vi "sv_Weighting Network Tolerances.vi"(9 "type or class":enum16{"Type 0 / Class 1", "Type 1 / Class 2"}(ring)=enum."Type 1 / Class 2", 10 "standard":enum16{"ANSI S1.4", "IEC 61672"}(ring), 11 "frequency [Hz]":dbl=1000.0 format="%.2f") -> (2 "low tolerance [dB]":dbl format="%.2f", 3 "high tolerance [dB]":dbl format="%.2f")   [LabVIEW 2017]
panel:
  in  "IEC 61672 tolerances [dB]":T1(array[cluster])=[{"frequency [Hz]"=[10.0, 12.589254117941675, 15.848931924611142, 19.952623149688797, 25.11886431509581, 31.622776601683793, 39.810717055349734, 50.11872336272725, 63.09573444801933, 79.43282347242817, 100.0, 125.89254117941675, 158.48931924611142, 199.52623149688807, 251.18864315095823, 316.22776601683796, 398.1071705534973, 501.18723362727246, 630.9573444801937, 794.3282347242822, 1000.0, 1258.9254117941675, 1584.893192461114, 1995.262314968881, 2511.886431509582, 3162.2776601683795, 3981.0717055349733, 5011.872336272725, 6309.573444801937, 7943.282347242822, 10000.0, 12589.254117941688, 15848.93192461114, 19952.62314968879], "high limit"=[3.0, 2.5, 2.0, 2.0, 2.0, 1.5, 1.0, 1.0, 1.0, 1.0, 1.0, 1.0, 1.0, 1.0, 1.0, 1.0, 1.0, 1.0, 1.0, 1.0, 0.7, 1.0, 1.0, 1.0, 1.0, 1.0, 1.0, 1.5, 1.5, 1.5, 2.0, 2.0, 2.5, 3.0], "low limit"=[-inf, -inf, -4.0, -2.0, -1.5, -1.5, -1.0, -1.0, -1.0, -1.0, -1.0, -1.0, -1.0, -1.0, -1.0, -1.0, -1.0, -1.0, -1.0, -1.0, -0.7, -1.0, -1.0, -1.0, -1.0, -1.0, -1.0, -1.5, -2.0, -2.5, -3.0, -5.0, -16.0, -inf]}, {"frequency [Hz]"=[10.0, 12.589254117941675, 15.848931924611142, 19.952623149688797, 25.11886431509581, 31.622776601683793, 39.810717055349734, 50.11872336272725, 63.09573444801933, 79.43282347242817, 100.0, 125.89254117941675, 158.48931924611142, 199.52623149688807, 251.18864315095823, 316.22776601683796, 398.1071705534973, 501.18723362727246, 630.9573444801937, 794.3282347242822, 1000.0, 1258.9254117941675, 1584.893192461114, 1995.262314968881, 2511.886431509582, 3162.2776601683795, 3981.0717055349733, 5011.872336272725, 6309.573444801937, 7943.282347242822, 10000.0, 12589.254117941688, 15848.93192461114, 19952.62314968879], "high limit"=[5.0, 5.0, 5.0, 3.0, 3.0, 3.0, 2.0, 2.0, 2.0, 2.0, 1.5, 1.5, 1.5, 1.5, 1.5, 1.5, 1.5, 1.5, 1.5, 1.5, 1.0, 1.5, 2.0, 2.0, 2.5, 2.5, 3.0, 3.5, 4.5, 5.0, 5.0, 5.0, 5.0, 5.0], "low limit"=[-inf, -inf, -inf, -3.0, -3.0, -3.0, -2.0, -2.0, -2.0, -2.0, -1.5, -1.5, -1.5, -1.5, -1.5, -1.5, -1.5, -1.5, -1.5, -1.5, -1.0, -1.5, -2.0, -2.0, -2.5, -2.5, -3.0, -3.5, -4.5, -5.0, -inf, -inf, -inf, -inf]}] caption="class" {"frequency [Hz]" format="%.2f"; "low limit" format="%.2f"; "high limit" format="%.2f"}
  in  "ANSI S1.4 tolerances [dB]":T1(array[cluster])=[{"frequency [Hz]"=[10.0, 12.59, 15.85, 19.95, 25.12, 31.5, 79.43, 100.0, 3981.07, 5011.87, 6309.57, 7943.28, 10000.0, 19952.62, 25118.86, 31622.78, 39810.72, 50118.72, 63095.73, 79432.82, 100000.0], "high limit"=[2.0, 2.0, 2.0, 2.0, 1.5, 1.0, 1.0, 0.7, 0.7, 1.0, 1.0, 1.0, 2.0, 2.0, 2.4, 2.8, 3.3, 4.1, 4.9, 5.1, 5.6], "low limit"=[-5.0, -4.0, -3.0, -2.0, -1.5, -1.0, -1.0, -0.7, -0.7, -1.0, -1.5, -2.0, -3.0, -3.0, -4.5, -6.2, -7.9, -9.3, -10.9, -12.2, -14.3]}, {"frequency [Hz]"=[10.0, 12.59, 15.85, 19.95, 25.12, 31.62, 39.81, 50.12, 3981.07, 5011.87, 6309.57, 7943.28, 10000.0, 12589.25, 15848.93, 19952.62, 25118.86, 31622.78, 39810.72, 50118.72, 63095.73, 79432.82, 100000.0], "high limit"=[4.0, 3.5, 3.0, 2.5, 2.0, 1.5, 1.5, 1.0, 1.0, 1.5, 1.5, 1.5, 2.0, 3.0, 3.0, 3.0, 3.5, 4.3, 5.0, 6.0, 6.9, 7.9, 8.9], "low limit"=[-4.0, -3.5, -3.0, -2.5, -2.0, -1.5, -1.5, -1.0, -1.0, -1.5, -2.0, -3.0, -4.0, -6.0, -7.4, -8.7, -9.6, -10.7, -11.7, -12.8, -13.9, -15.2, -16.8]}] caption="type" {"frequency [Hz]" format="%.2f"; "low limit" format="%.2f"; "high limit" format="%.2f"}
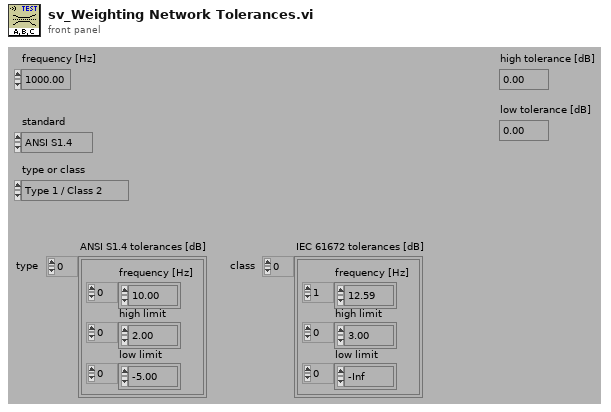
[diagram p1: front panel]
types:
  T1 = cluster{"frequency [Hz]":dbl[], "high limit":dbl[], "low limit":dbl[]}[]
  T2 = cluster{"frequency [Hz]":dbl[], "high limit":dbl[], "low limit":dbl[]}
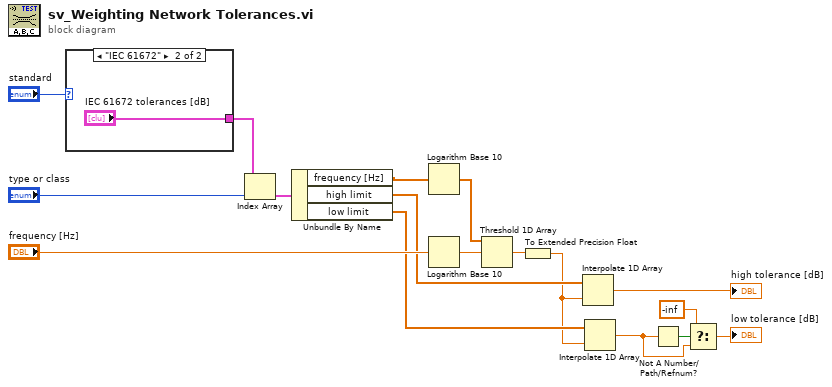
[diagram p0: block diagram]
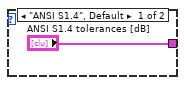
[diagram p2: hidden frame]
diagram:
  n1 = case shown="\"IEC 61672\"" "standard" {
    tunnel: ["ANSI S1.4 tolerances [dB]" "IEC 61672 tolerances [dB]"] -> w17
    frame "ANSI S1.4", Default {
    }
    frame "IEC 61672" {
    }
  }
  n2 = Index Array(array=w17, index="type or class") -> (element=w16:T2)
  n3 = Unbundle By Name(w16) -> ("frequency [Hz]"=w11:dbl[], "high limit"=w13:dbl[], "low limit"=w12:dbl[])
  n4 = Logarithm Base 10(1:w11) -> (0:w1:dbl[])
  n5 = Logarithm Base 10(1:"frequency [Hz]") -> (0:w2:dbl)
  n6 = Threshold 1D Array(2:w2, 3:w1) -> (0:w10:dbl)  [unwired: 1 in]
  n7 = To Extended Precision Float(1:w10) -> (0:w9:ext)
  n8 = Interpolate 1D Array(1:w9, 2:w13) -> (0:→"high tolerance [dB]":dbl)
  n9 = Interpolate 1D Array(1:w9, 2:w12) -> (0:w3:dbl)
  n10 = Not A Number/Path/Refnum?(number/path/refnum=w3) -> (NaN/Path/Refnum?=w4:bool)
  n11 = Select(t=-inf ("y"), s=w4, f=w3) -> (s? t:f=→"low tolerance [dB]":dbl)
